vi "Save_current_setup.vi"(3 "Save New File?":bool, 4 "jobDirectory":path, 5 "Setup File Type":T1) -> (0 "Cancelled?":bool, 1 "Saved filepath":path, 2 "Current Setup":path)   [LabVIEW 2022 SP3]
uses:
  File/Setup_Filetype.ctl
  0946215b-995a-a842-9bcf-0b3b3613d8fb.vi
  Data_plotting_vis/Results_plotter_Global.vi
panel:
  out "Existing Setup names":string[](array[string])
  in  "New Setup filename":string
  in  "Cancel Button":bool
  in  "OK":bool
  # "To re-use an existing filename, click on a name in the array on the left, or else type a new one"
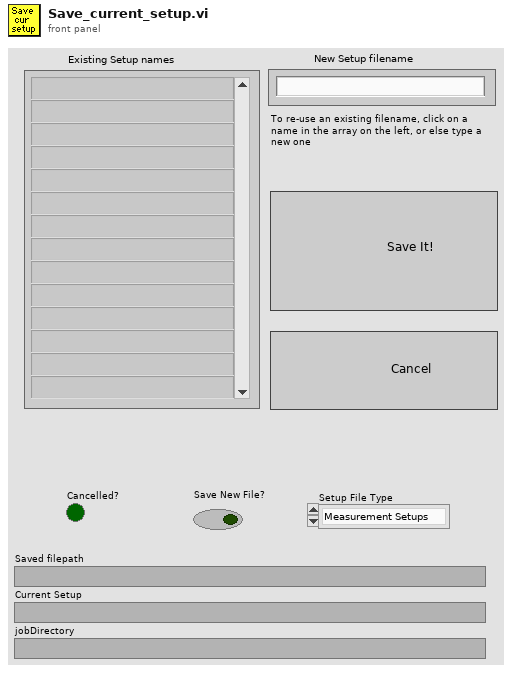
[diagram p1: front panel]
types:
  T1 = typedef "Setup_Filetype.ctl" = enum16{"Measurement Setups", "Calibration Setups", "General", "Results File Plotter Setups", "Speed Calib Tweaks"}
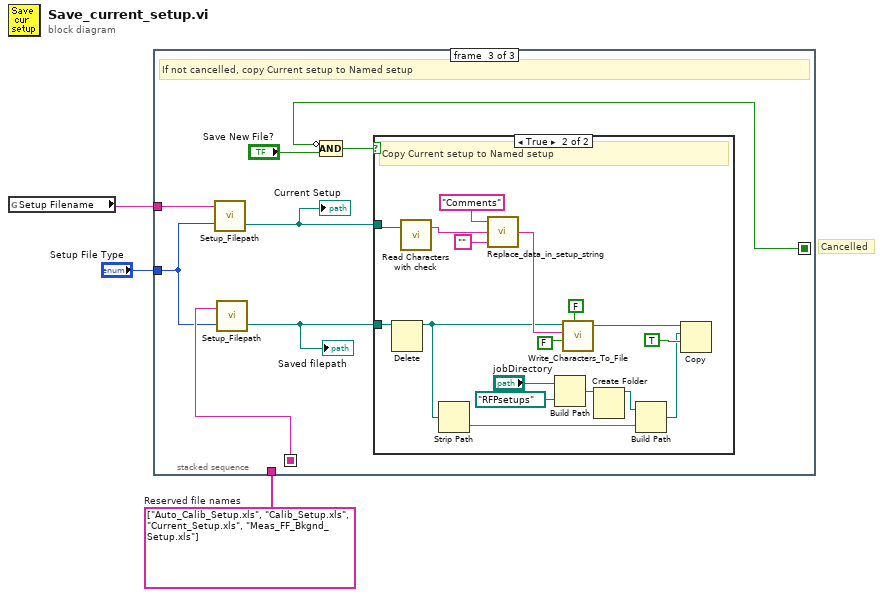
[diagram p0: block diagram]
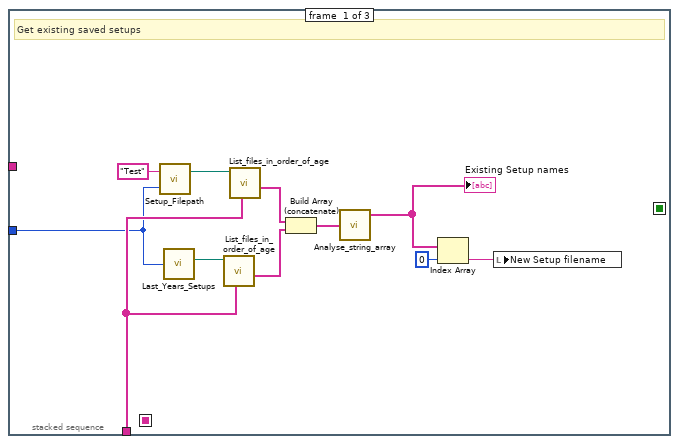
[diagram p2: hidden frame]
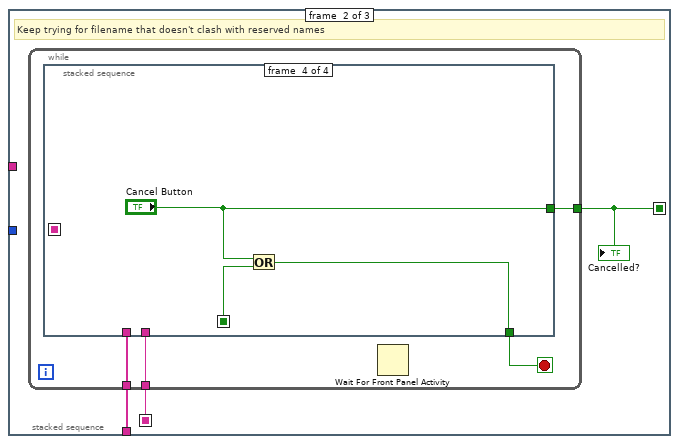
[diagram p3: hidden frame]
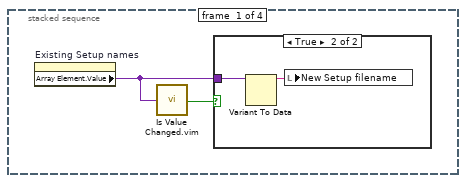
[diagram p4: hidden frame]
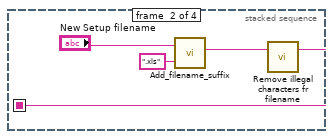
[diagram p6: hidden frame]
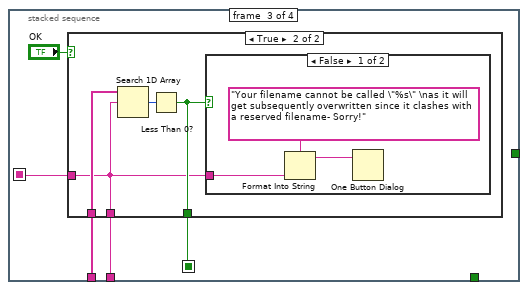
[diagram p7: hidden frame]
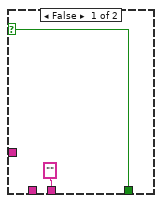
[diagram p8: hidden frame]
diagram:
  w3 = string[] ["Auto_Calib_Setup.xls", "Calib_Setup.xls", "Current_Setup.xls", "Meas_FF_Bkgnd_Setup.xls"]  # Reserved file names
  # "Cancelled"
  n1 = global read "Results_plotter_Global.vi" "Setup Filename"() -> (w1:string)
  n2 = stacked-sequence {
    seq-local: [_ w17 _] -> [_ _ w50]
    seq-local: [_ w16 _] -> [_ _ w54]
    tunnel: w3 -> [w12 w15 _]
    tunnel: "Setup File Type" -> [w6 _ w48]
    tunnel: w1 -> [_ _ w47]
    frame #0 {
      # "Get existing saved setups"
      n3 = call "Setup_Filepath.vi"("Setup File Type"=w6, "Filename in"="Test") -> ("Directory"=w10:path)  [unwired: 1 out]
      n4 = call "Last_Years_Setups.vi"("Setup File Type"=w6) -> ("Directory"=w11:path)
      n5 = call "List_files_in_order_of_age.vi"("Files to Hide"=w12, "Folder"=w11) -> ("file names"=w8:string[])  [unwired: 9 in]
      n6 = call "List_files_in_order_of_age.vi"("Files to Hide"=w12, "Folder"=w10) -> ("file names"=w9:string[])  [unwired: 9 in]
      n7 = Build Array (concatenate)(w9, w8) -> (w5:string[])
      n8 = call "Analyse_string_array.vi"("String array"=w5) -> ("Unique strings"=w4:string[])  [unwired: 1 in, 1 out]
      "Existing Setup names" <- w4
      n9 = Index Array(array=w4, index=0) -> (element=w13:string)
      n10 = local write "New Setup filename"(w13) -> ()
    }
    frame #1 {
      # "Keep trying for filename that doesn't clash with reserved names"
      n11 = while {
        tunnel: [w21] -> w17
        tunnel: [w19] -> w16
        tunnel: w15 -> [w18]
        stop <- w20 stop-if-true
        n12 = stacked-sequence {
          seq-local: [_ w26 _ _] -> [_ _ w34 _]
          seq-local: [_ _ w32 _] -> [_ _ _ w46]
          tunnel: [_ _ w33 _] -> w21
          tunnel: [_ _ _ w45] -> w20
          tunnel: [_ _ _ "Cancel Button"] -> w19
          tunnel: w18 -> [_ _ w30 _]
          frame #0 {
            n13 = property on="Existing Setup names" class="Arr (strict)"() -> ("Array Element.Value"=w23:variant)  [unwired: 2 in, 2 out]
            n14 = call "Is Value Changed.vim"("value"=w23) -> ("changed or first call?"=w22:bool)
            n15 = case shown="True" w22 {
              tunnel: w23 -> [_ w24]
              frame False {
              }
              frame True {
                n16 = Variant To Data(Variant=w24) -> (data=w25:string)  [unwired: 2 in, 1 out]
                n17 = local write "New Setup filename"(w25) -> ()
              }
            }
          }
          frame #1 {
            n18 = call "Add_filename_suffix.vi"("Filename"="New Setup filename", "Suffix to add"=".xls") -> ("Filename out"=w27:string)  [unwired: 3 out]
            n19 = call "Remove illegal characters fr filename.vi"("Filename In"=w27) -> ("Cleaned Filename"=w26:string)  [unwired: 2 in]
          }
          frame #2 {
            n20 = case shown="True" "OK" {
              selector: "OK" -> [w35 _]
              tunnel: w34 -> [_ w37]
              tunnel: [w35 w38] -> w32
              tunnel: ["" ("File name only") w37] -> w33
              tunnel: w30 -> [_ w40]
              frame False {
              }
              frame True {
                n21 = Search 1D Array(1D array=w40, element=w37) -> (index of element=w39:i32)  [unwired: 1 out]
                n22 = Less Than 0?(x=w39) -> (x < 0?=w38:bool)
                n23 = case shown="False" w38 {
                  tunnel: w37 -> [w42 _]
                  frame False {
                    n24 = Format Into String(format string="Your filename cannot be called \"%s\" \nas it will get subsequently overwritten since it clashes with a reserved filename- Sorry!", w42) -> (resulting string=w41:string)  [unwired: 2 in, 1 out]
                    n25 = One Button Dialog(message=w41) -> ()  [unwired: 2 out]
                  }
                  frame True {
                  }
                }
              }
            }
          }
          frame #3 {
            n26 = Or(x="Cancel Button", y=w46) -> (x .or. y?=w45:bool)
          }
        }
        n27 = Wait For Front Panel Activity() -> ()  [unwired: 3 in, 1 out]
      }
      "Cancelled?" <- w16
    }
    frame #2 {
      # "If not cancelled, copy Current setup to Named setup"
      n28 = call "Setup_Filepath.vi"("Setup File Type"=w48, "Filename in"=w47) -> ("Filename Out"=w51:path)  [unwired: 1 out]
      "Current Setup" <- w51
      n29 = call "Setup_Filepath.vi"("Setup File Type"=w48, "Filename in"=w50) -> ("Filename Out"=w49:path)  [unwired: 1 out]
      "Saved filepath" <- w49
      n30 = Compound Arithmetic op=AND(invert w54, "Save New File?") -> (w52:bool)
      n31 = case shown="True" w52 {
        tunnel: w51 -> [_ w56]
        tunnel: w49 -> [_ w71]
        frame False {
        }
        frame True {
          # "Copy Current setup to Named setup"
          n32 = Delete(path (use dialog)=w71) -> (deleted path=w62:path)  [unwired: 4 in, 2 out]
          n33 = call "Read Characters with check.vi"("file (use dialog)"=w56) -> ("Read String"=w55:string)  [unwired: 1 in, 1 out]
          n34 = Strip Path(path=w62) -> (name=w61:string)  [unwired: 1 out]
          n35 = call "Replace_data_in_setup_string.vi"("New data string"="", "Input string"=w55, "Variable name"="Comments") -> ("Appended string"=w66:string)
          n36 = Build Path(base path="jobDirectory", name or relative path=path "RFPsetups") -> (appended path=w58:path)
          n37 = call "Write_Characters_To_File.vi"("file path (dialog if empty)"=w62, "advisory dialog? (display:T)"=FALSE, "character string"=w66, "append to file? (new file:F)"=FALSE) -> ("pathOut"=w65:path)  [unwired: 1 in, 3 out]
          n38 = Create Folder(path (use dialog)=w58) -> (created path=w57:path)  [unwired: 2 in, 2 out]
          n39 = Build Path(base path=w57, name or relative path=w61) -> (appended path=w60:path)
          n40 = Copy(9:TRUE ("overwrite (F)"), 10:w60, 11:w65) -> ()  [unwired: 2 in, 3 out]
        }
      }
    }
  }
